vi "tolerance calculator.vi"(8 "error in (no error)":errorcluster, 10 "Set point":dbl, 11 "Abs value":dbl) -> (0 "error out":errorcluster, 3 "output cluster":T1)   [LabVIEW 2019]
panel:
  in  "ALIMENTATORE VARIAC":T2={"STATO"={"Comunicazione"=FALSE, "Abilitato"=FALSE, "RUNNING"=FALSE, "ALLARME"=FALSE, "FINE RAMPA"=FALSE}, "START\\STOP"={"START"=FALSE, "STOP"=FALSE}, "SETPOINT"={"TENSIONE [V]"=0.0, "Rampa tensione"=0.0, "PID V"=FALSE, "PID F"=FALSE, "SET V F"=FALSE}, "connetti"={"Comunicazione"=FALSE, "Connetti"=FALSE, "Disconnetti"=FALSE}, "Stato config"={"RPM"=0.0, "Vnom"=0.0, "HZnom"=0.0, "Inom"=0.0, "kWnom"=0.0, "TipoMot."=0.0}, "Controlli"={"Trampa[s]"=10.0, "Stato rampa"=10.0, "Inverti senso di rotazione"=FALSE}, "Config"=FALSE} {"Controlli"."Trampa[s]" min=0.1; "SETPOINT"."Rampa tensione" scale=0.0..500.0}
  # "~ ALIMENTATORE VARIAC~"
  # "CONNESSIONE..."
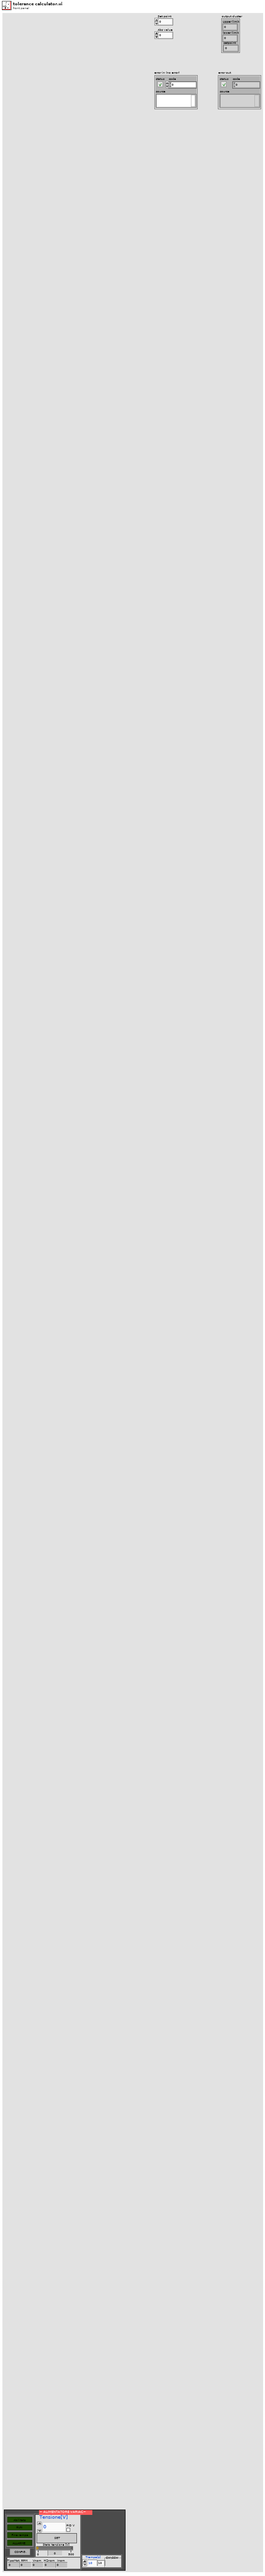
[diagram p1: front panel]
types:
  T1 = cluster{"upper limit":dbl, "lower limit":dbl, "setpoint":dbl}
  T2 = cluster{"STATO":cluster{"Comunicazione":bool, "Abilitato":bool, "RUNNING":bool, "ALLARME":bool, "FINE RAMPA":bool}, "START\\STOP":cluster{"START":bool, "STOP":bool}, "SETPOINT":cluster{"TENSIONE [V]":dbl, "Rampa tensione":dbl, "PID V":bool, "PID F":bool, "SET V F":bool}, "connetti":cluster{"Comunicazione":bool, "Connetti":bool, "Disconnetti":bool}, "Stato config":cluster{"RPM":dbl, "Vnom":dbl, "HZnom":dbl, "Inom":dbl, "kWnom":dbl, "TipoMot.":dbl}, "Controlli":cluster{"Trampa[s]":dbl, "Stato rampa":dbl, "Inverti senso di rotazione":bool}, "Config":bool}
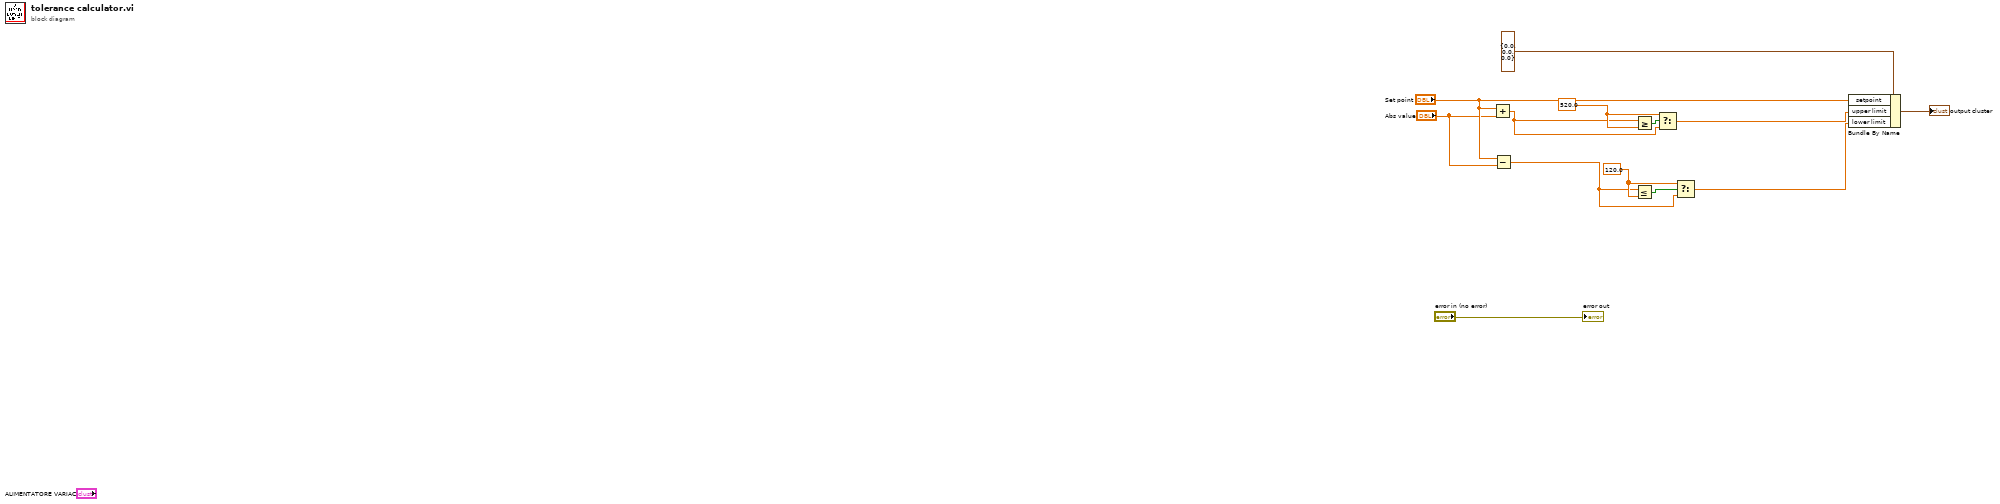
[diagram p0: block diagram]
diagram:
  w4 = 120.0 ("y")
  w7 = 520.0 ("y")
  n1 = Add(x="Set point", y="Abs value") -> (x+y=w6:dbl)
  n2 = Subtract(x="Set point", y="Abs value") -> (x-y=w3:dbl)
  n3 = Less Or Equal?(x=w3, y=w4) -> (x <= y?=w1:bool)
  n4 = Greater Or Equal?(x=w6, y=w7) -> (x >= y?=w8:bool)
  n5 = Select(t=w7, s=w8, f=w6) -> (s? t:f=w5:dbl)
  n6 = Select(t=w4, s=w1, f=w3) -> (s? t:f=w2:dbl)
  n7 = Bundle By Name(cluster=T1 {"upper limit"=0.0, "lower limit"=0.0, "setpoint"=0.0}, "setpoint"="Set point", "upper limit"=w5, "lower limit"=w2) -> (→"output cluster":T1)
  "error out" <- "error in (no error)"
